vi "Chroma_PowerSupply_ON.vi"(8 "错误输入（无错误）":errorcluster, 11 "VISA资源名称":refnum<visa-resource-name>="COM1") -> (0 "错误输出":errorcluster, 3 "VISA资源名称输出":refnum<visa-resource-name>)   [LabVIEW 2012]
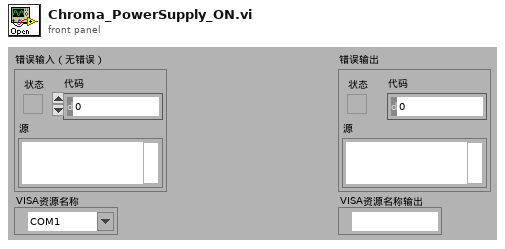
[diagram p1: front panel]
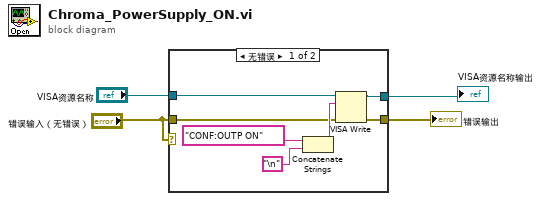
[diagram p0: block diagram]
diagram:
  n1 = case shown="无错误" "错误输入（无错误）" {
    tunnel: "VISA资源名称" -> [w9 w13]
    tunnel: "错误输入（无错误）" -> [w8 w12]
    tunnel: [w7 w13] -> w3
    tunnel: [w6 w12] -> w2
    frame No Error {
      n2 = Concatenate Strings("CONF:OUTP ON" ("写入缓冲区"), "\n") -> (w10:string)
      n3 = VISA Write(VISA resource name=w9, write buffer=w10, error in (no error)=w8) -> (VISA resource name out=w7:refnum<visa-resource-name>, error out=w6:errorcluster)  [unwired: 1 out]
    }
    frame Error {
    }
  }
  "错误输出" <- w2
  "VISA资源名称输出" <- w3
